vi "Start Jl Server, Init LV client, check comm.vi"(0 "endpoint":string, 5 "Julia user functions script":path=path "dummy.jl", 9 "request":string, 11 "error in (no error)":errorcluster) -> (2 "LV client state":T1, 3 "JL server state":T1, 4 "zmq_context out":refnum<class "zmq_context.lvclass">, 6 "zmq_socket out":refnum<class "zmq_socket.lvclass">, 8 "response":string, 10 "script return code (0)":i32, 12 "jl-script file path":path, 13 "tmp file path":path, 14 "timeout?":bool, 15 "error out":errorcluster)   [LabVIEW 2018, in "LV-0mq-Julia_roundtrip-lib.lvlib" / "LV2Julia_core.lvlib"]
uses:
  LV2Julia_core.lvlib
  Server or client state.ctl
  <vilib>/addons/zeromq/zmq_socket.lvclass
  <vilib>/addons/zeromq/zmq_context.lvclass
  ZMQ timeouts global.vi
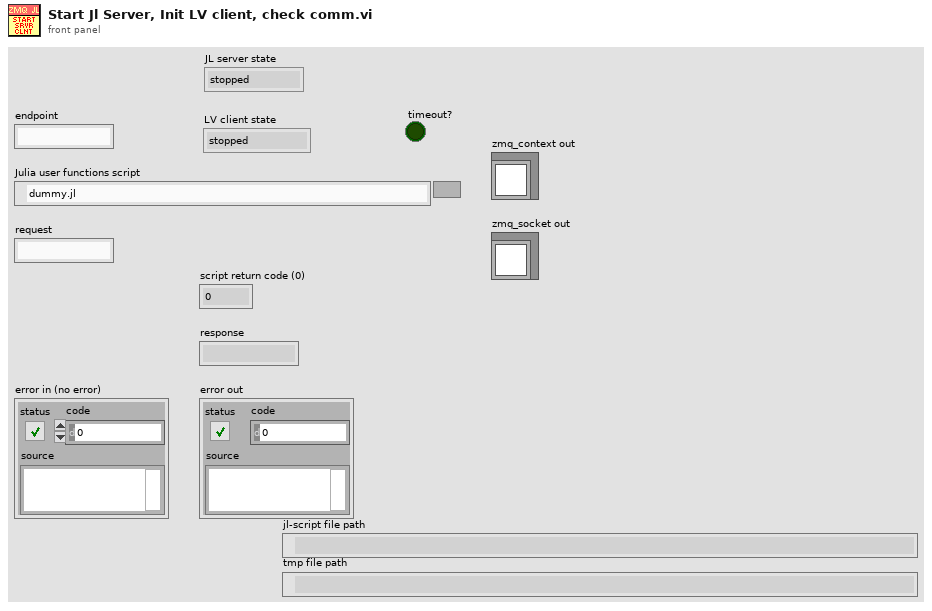
[diagram p1: front panel]
types:
  T1 = typedef "LV-0mq-Julia_roundtrip-lib.lvlib/LV2Julia_core.lvlib/Server or client state.ctl" = enum16{"stopped", "running", "unknown"}
  T2 = typedef "LV-0mq-Julia_roundtrip-lib.lvlib/LV2Julia_core.lvlib/ZMQ timeouts.ctl" = cluster{"SNDTIMEO":i32, "RCVTIMEO":i32}
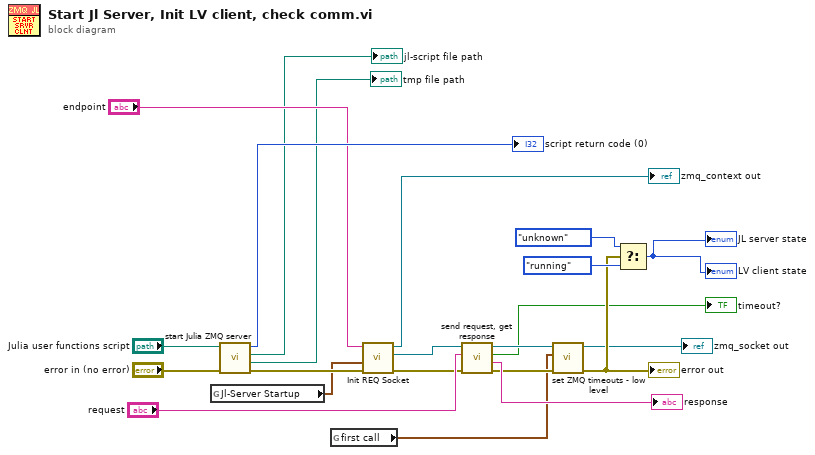
[diagram p0: block diagram]
diagram:
  n1 = global read "ZMQ timeouts global.vi" "Jl-Server Startup"() -> (w3:T2)
  n2 = call "start Julia ZMQ server.vi"("error in (no error)"="error in (no error)", "Julia user functions script"="Julia user functions script") -> ("error out"=w18:errorcluster, "tmp file out"=→"tmp file path":path, "jl-script file out"=→"jl-script file path":path, "return code"=→"script return code (0)":i32)  [unwired: 6 in]
  n3 = global read "ZMQ timeouts global.vi" "first call"() -> (w4:T2)
  n4 = call "Init REQ Socket.vi"("error in (no error)"=w18, "ZMQ new Timeouts in"=w3, "endpoint"="endpoint") -> ("error out"=w12:errorcluster, "socket out"=w15:refnum<class "zmq_socket.lvclass">, "zmq_context out"=→"zmq_context out":refnum<class "zmq_context.lvclass">)  [unwired: 5 in, 1 out]
  n5 = call "send request, get response.vi"("error in (no error)"=w12, "request"="request", "zmq_socket in"=w15) -> ("error out"=w9:errorcluster, "response"=→"response":string, "timeout?"=→"timeout?":bool, "zmq_socket out"=w7:refnum<class "zmq_socket.lvclass">)  [unwired: 4 in, 1 out]
  n6 = call "set ZMQ timeouts - low level.vi"("error in (no error)"=w9, "ZMQ new Timeouts in"=w4, "zmq_socket in"=w7) -> ("error out"=w8:errorcluster, "zmq_socket out"=→"zmq_socket out":refnum<class "zmq_socket.lvclass">)  [unwired: 6 in, 1 out]
  "error out" <- w8
  n7 = Select(t=Server_or_client_state."unknown" ("Server state"), s=w8, f=Server_or_client_state."running") -> (s? t:f=→"JL server state" →"LV client state":T1)
